vi "Unshow Controls as Icons.vi"(8 "error in":errorcluster, 10 "Save VI?":bool, 11 "vi path":path) -> (0 "error out":errorcluster)   [LabVIEW 2023]
uses:
  <vilib>/Utility/traverseref.llb/TRef TravTarget.ctl
  <vilib>/Utility/traverseref.llb/VI Scripting - Traverse.lvlib
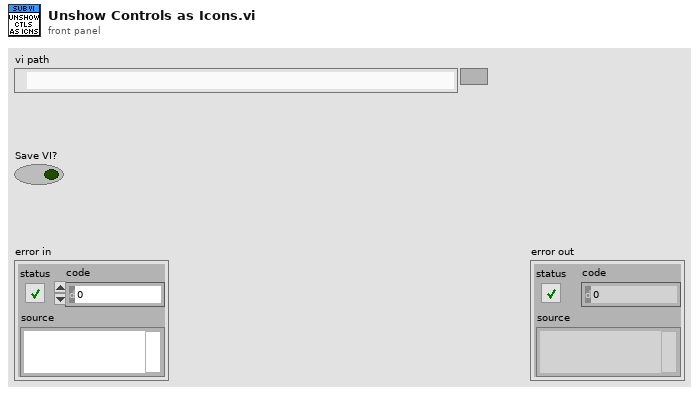
[diagram p1: front panel]
types:
  T1 = typedef "TRef TravTarget.ctl" = enum16{"FP", "BD", "Other"}
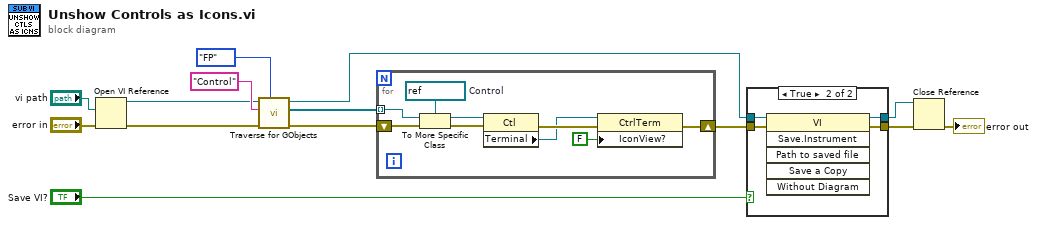
[diagram p0: block diagram]
diagram:
  n1 = Open VI Reference(vi path="vi path", error in (no error)="error in") -> (vi reference=w7:refnum<vi>, error out=w13:errorcluster)  [unwired: 4 in]
  n2 = call <vilib>:"Traverse for GObjects.vi"("Traverse Target"=TRef_TravTarget."FP", "error in (no error)"=w13, "Class Name"="Control", "VI Refnum"=w7) -> ("error out"=w12:errorcluster, "References"=w9:refnum<vi>[], "dup VI Refnum"=w5:refnum<vi>)  [unwired: 4 in, 1 out]
  n3 = for {
    tunnel: w9 -> [w20] mode=indexing
    shift-right: [w15] -> w6
    shift-left: w12 -> [w23]
    w19 = refnum<vi> refnum  # Control
    n4 = To More Specific Class(target class=w19, reference=w20, error in=w23) -> (specific class reference=w18:refnum<vi>, error out=w22:errorcluster)
    n5 = property class="Ctl"(reference=w18, error in=w22) -> (error out=w21:errorcluster, "Terminal"=w17:refnum<vi>)  [unwired: 1 out]
    n6 = property class="CtrlTerm"(reference=w17, error in=w21, "IconView?"=FALSE ("Icon View?")) -> (error out=w15:errorcluster)  [unwired: 1 out]
  }
  n7 = case shown="True" "Save VI?" {
    tunnel: w6 -> [w25 w29]
    tunnel: [w25 w28] -> w3
    tunnel: [w24 w27] -> w2
    tunnel: w5 -> [w24 w26]
    frame False {
    }
    frame True {
      n8 = invoke class="VI" method="Save.Instrument"(reference=w26, error in=w29) -> (reference out=w27:refnum<vi>, error out=w28:errorcluster)  [unwired: 4 in, 4 out]
    }
  }
  n9 = Close Reference(reference=w2, error in (no error)=w3) -> (error out=→"error out":errorcluster)
